vi "Calibrate LCVR.vi"() -> ()   [LabVIEW 2012]
uses:
  <vilib>/DAQmx/write.llb/DAQmx Write (Analog DBL 1Chan 1Samp).vi
  <vilib>/DAQmx/write.llb/DAQmx Write (Digital Bool 1Line 1Point).vi
  <vilib>/DAQmx/write.llb/DAQmx Write (Digital 1D Bool 1Chan 1Samp).vi
  <vilib>/DAQmx/create/channels.llb/DAQmx Create Channel (DO-Digital Output).vi
  <vilib>/DAQmx/create/channels.llb/DAQmx Create Channel (AO-Voltage-Basic).vi
  <vilib>/DAQmx/miscellaneous.llb/DAQmx Fill In Error Info.vi
  <userlib>/metrolib-x86/metrolib-x86.lvlib
panel:
  in  "Ouput Path":path
  in  "Focus":bool
  out "Contrast":cluster{dbl[], dbl[]}(graph)
  out "Image":dbl[][](graph)
  out "Current V":dbl
  out "step":i32
  out "Delta V":dbl
  in  "Steps":i32=40
  in  "Max V":dbl=8.0
  in  "Min V":dbl
  in  "Exposure (ms)":dbl=50.0
  in  "stop":bool
  in  "Sweep":bool
  out "Error Out":errorcluster
  in  "SLM RO":u8 max=38
  # "LCVR Calibration Tool"
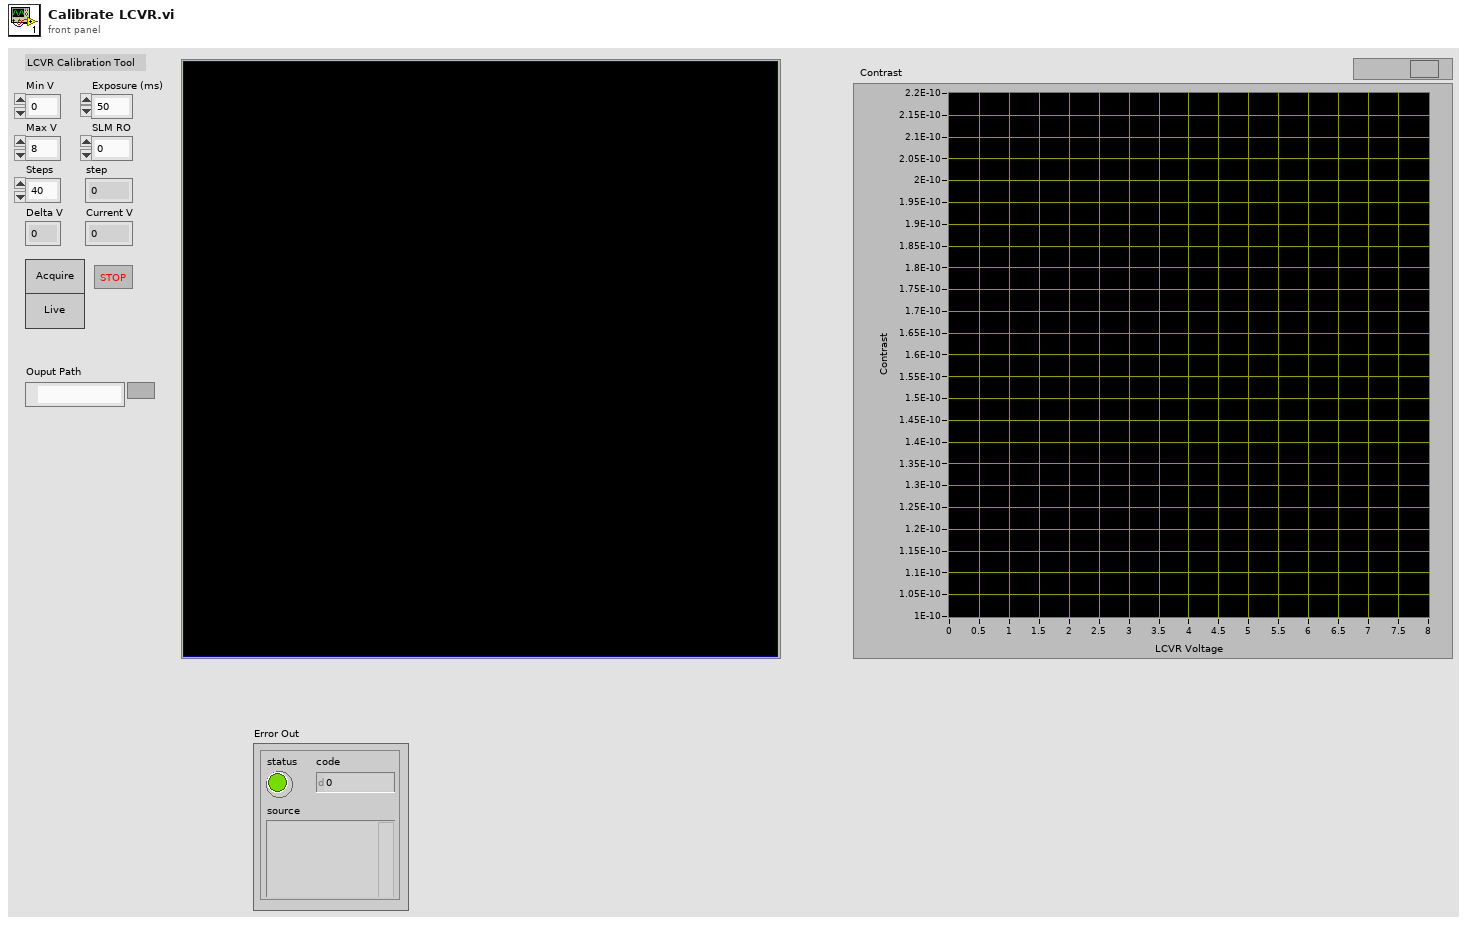
[diagram p1: front panel]
types:
  T1 = cluster{"Mode":u32, "Polarity":u32, "Period":dbl, "Delay":dbl}
  T2 = cluster{"Horizontal Offset":i32, "Vertical Offset":i32, "Horizontal Width":i32, "Vertical Width":i32}
  T3 = cluster{"height":u32, "width":u32, "datatype":u32}
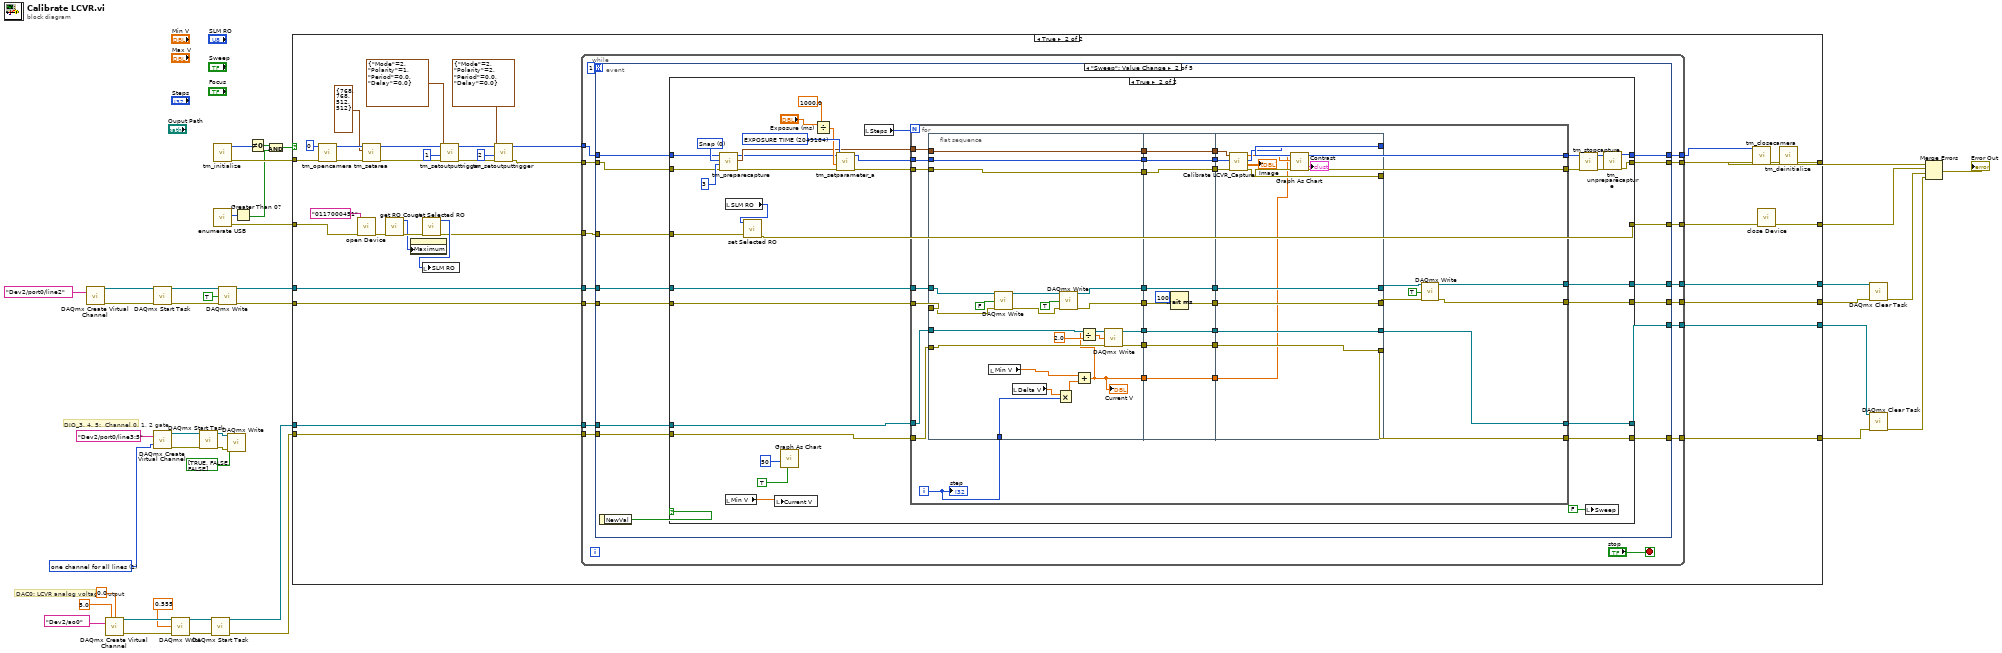
[diagram p0: block diagram]
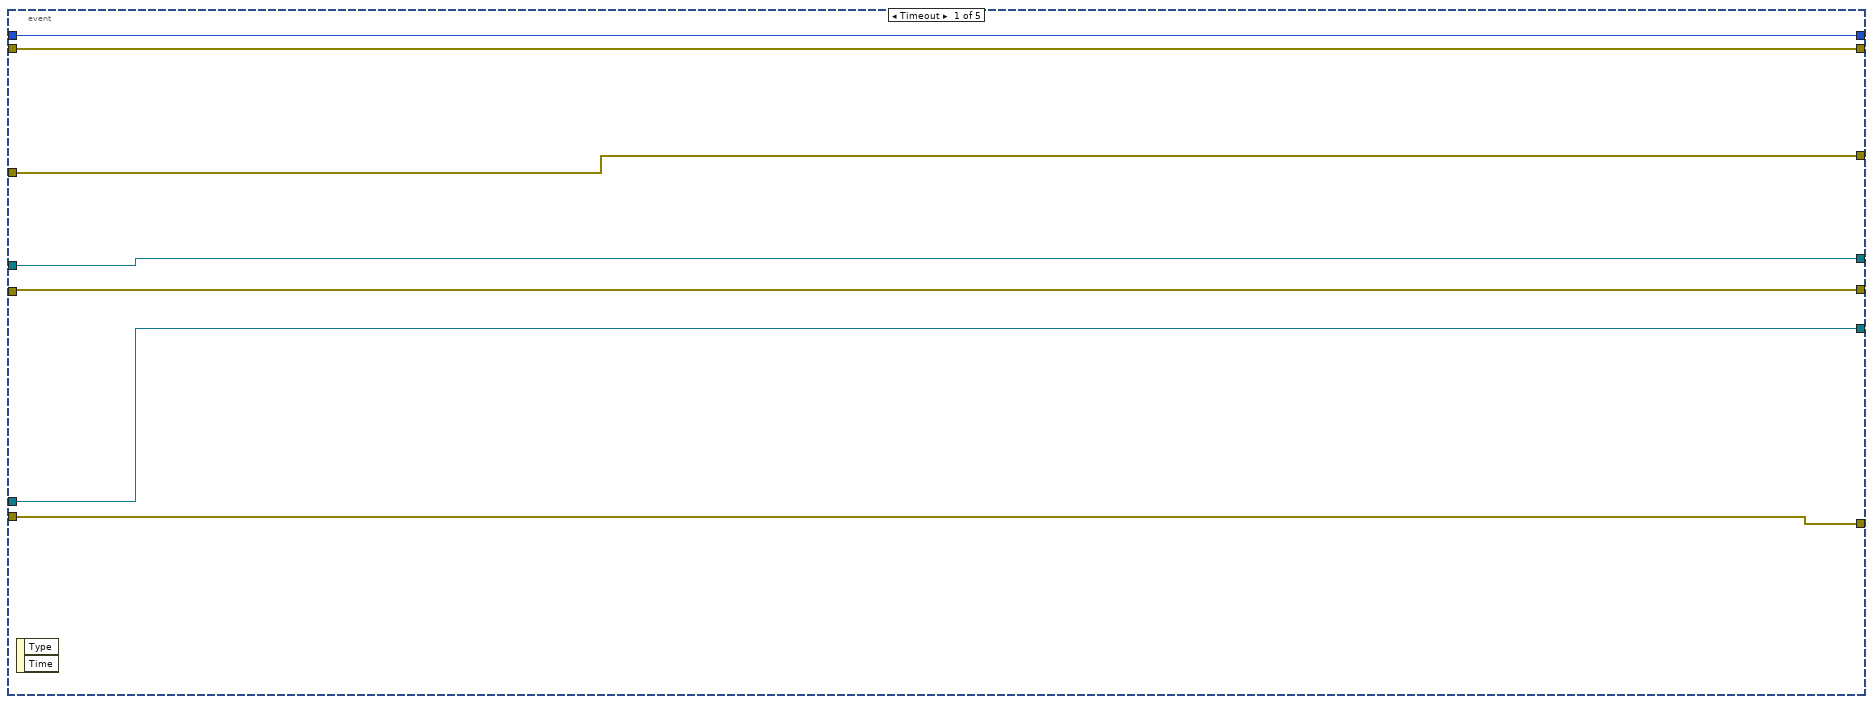
[diagram p3: hidden frame]
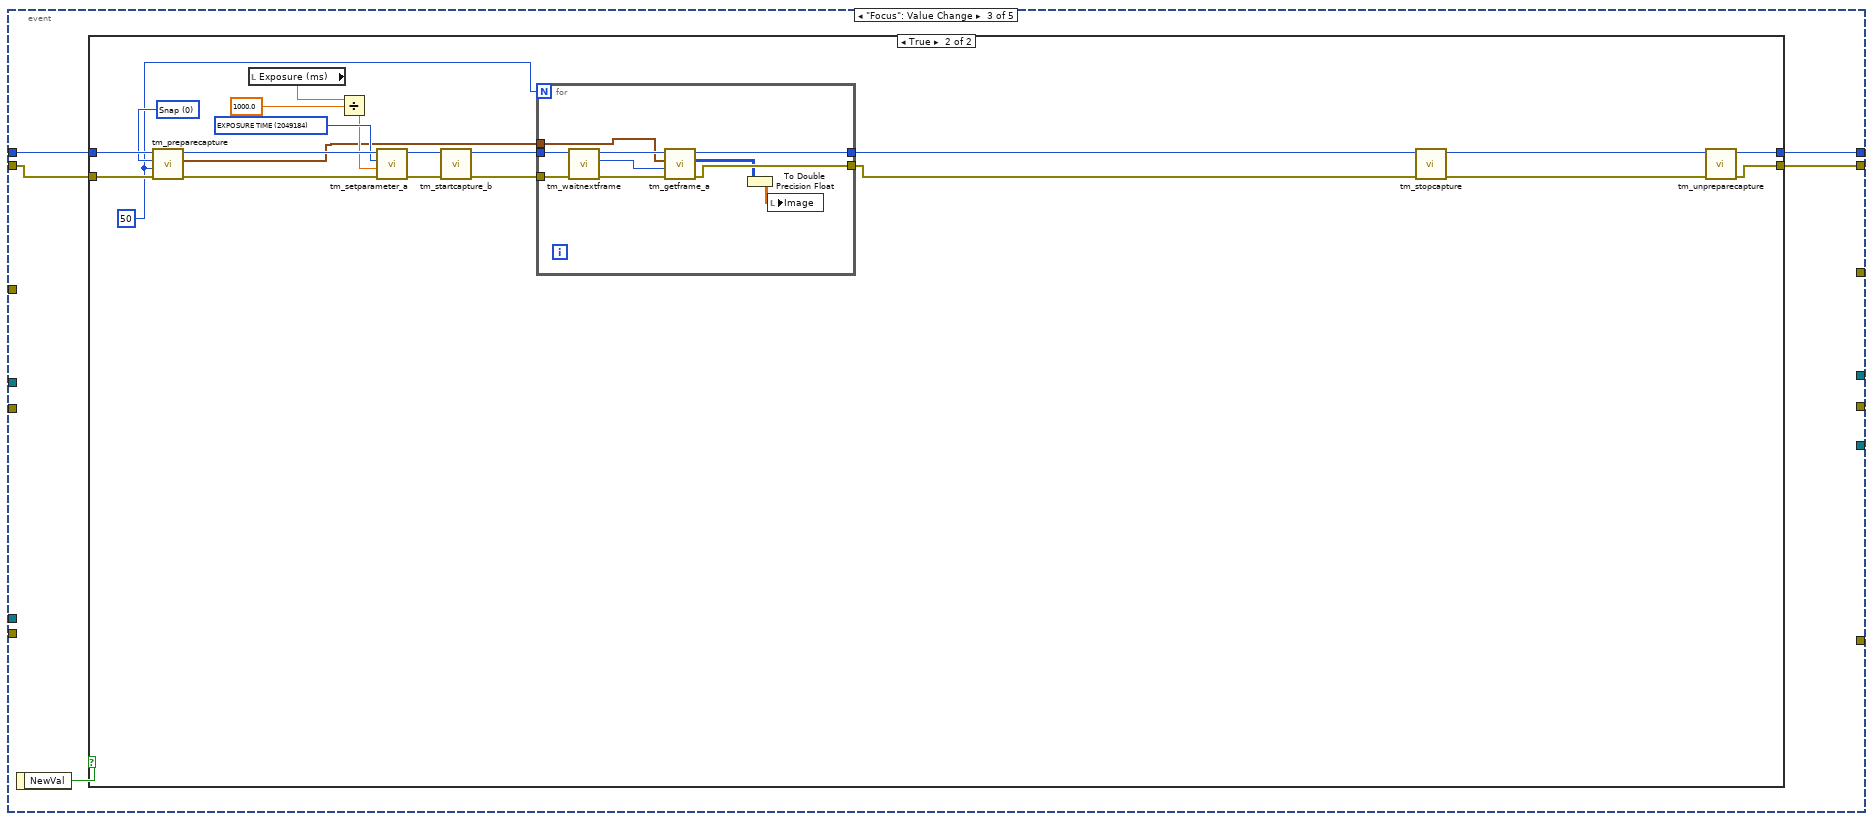
[diagram p5: hidden frame]
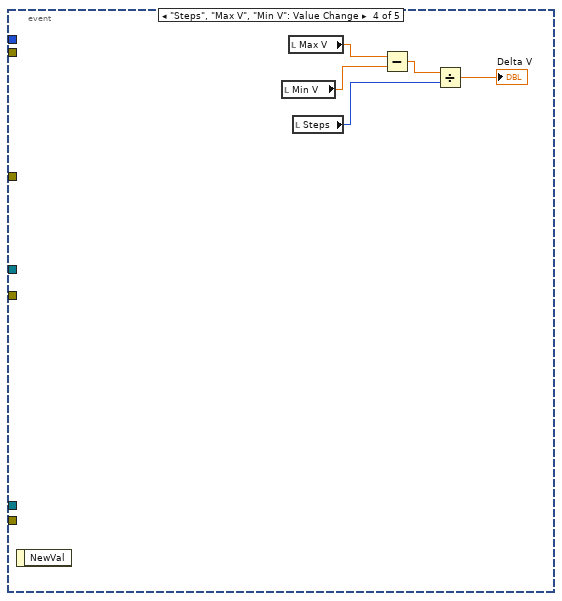
[diagram p7: hidden frame]
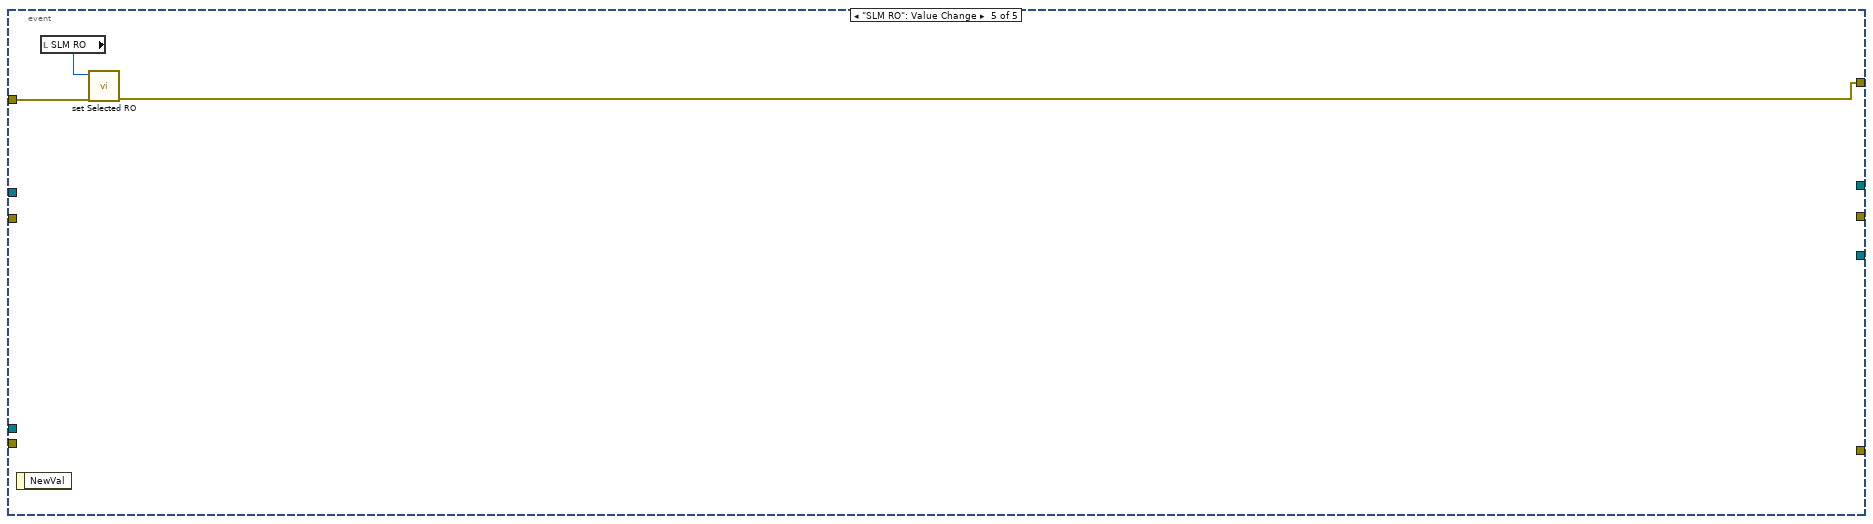
[diagram p8: hidden frame]
diagram:
  w30 = 1 items=["one channel for each line", "one channel for all lines"] ("line grouping")
  # "DAC0: LCVR analog voltage output"
  # "DIO_3, 4, 5:  Channel 0, 1, 2 gate"
  n1 = call-poly <vilib>:"DAQmx Create Virtual Channel.vi"("lines"=tag "Dev2/port0/line2") -> ("task out"=w26:refnum<k21>, "error out"=w25:errorcluster)  [unwired: 13 in]
  n2 = call-poly <vilib>:"DAQmx Create Virtual Channel.vi"("maximum value"=5.0, "minimum value"=0.0, "physical channels"=tag "Dev2/ao0") -> ("task out"=w8:refnum<k21>, "error out"=w7:errorcluster)  [unwired: 11 in]
  n3 = call <vilib>:"DAQmx Start Task.vi"("task/channels in"=w26, "error in"=w25) -> ("task out"=w24:refnum<k21>, "error out"=w23:errorcluster)  [unwired: 12 in]
  n4 = call-poly <vilib>:"DAQmx Create Virtual Channel.vi"("lines"="Dev2/port0/line3:5", "line grouping"=w30) -> ("task out"=w29:refnum<k21>, "error out"=w28:errorcluster)  [unwired: 12 in]
  n5 = call-poly <vilib>:"DAQmx Write.vi"("task/channels in"=w8, "data"=0.555, "error in"=w7) -> ("task out"=w12:refnum<k21>, "error out"=w11:errorcluster)  [unwired: 10 in, 1 out]
  n6 = call <vilib>:"DAQmx Start Task.vi"("task/channels in"=w29, "error in"=w28) -> ("task out"=w21:refnum<k21>, "error out"=w14:errorcluster)  [unwired: 12 in]
  n7 = call <vilib>:"DAQmx Start Task.vi"("task/channels in"=w12, "error in"=w11) -> ("task out"=w4:refnum<k21>, "error out"=w3:errorcluster)  [unwired: 12 in]
  n8 = call <userlib>:"tm_initialize.vi"() -> ("error out"=w39:errorcluster, "Number Of Cameras"=w40:u32)  [unwired: 8 in, 2 out]
  n9 = call <userlib>:"enumerate USB.vi"() -> ("error out"=w38:errorcluster, "function return"=w41:i16)  [unwired: 9 in, 1 out]
  n10 = call-poly <vilib>:"DAQmx Write.vi"("task/channels in"=w24, "data"=TRUE, "error in"=w23) -> ("task out"=w19:refnum<k21>, "error out"=w18:errorcluster)  [unwired: 10 in, 1 out]
  n11 = call-poly <vilib>:"DAQmx Write.vi"("task/channels in"=w21, "data"=bool[] [TRUE, FALSE, FALSE], "error in"=w14) -> ()  [unwired: 10 in, 3 out]
  n12 = Greater Than 0?(x=w41) -> (x > 0?=w35:bool)
  n13 = Not Equal To 0?(x=w40) -> (x != 0?=w37:bool)
  n14 = And(x=w37, y=w35) -> (x .and. y?=w36:bool)
  n15 = case shown="True" w36 {
    tunnel: w39 -> [w47 w82]
    tunnel: w38 -> [w46 w76]
    tunnel: [w47 w73] -> w33
    tunnel: [w46 w71] -> w32
    tunnel: w19 -> [w45 w59]
    tunnel: w18 -> [w44 w58]
    tunnel: [w44 w57] -> w17
    tunnel: [w45 w56] -> w16
    tunnel: w4 -> [w43 w55]
    tunnel: w3 -> [w42 w54]
    tunnel: [w43 w53] -> w2
    tunnel: [w42 w52] -> w1
    frame False {
    }
    frame True {
      n16 = call <userlib>:"tm_opencamera.vi"("error in (no error)"=w82, "Camera Index"=u32 0) -> ("error out"=w70:errorcluster, "Handle out"=w69:u32)  [unwired: 7 in, 1 out]
      n17 = call <userlib>:"open Device.vi"("error in (no error)"=w76, "identifier"="0117000451") -> ("error out"=w77:errorcluster)  [unwired: 8 in, 1 out]
      n18 = call <userlib>:"tm_setarea.vi"("error in (no error)"=w70, "Sub Region"=T2 {"Horizontal Offset"=768, "Vertical Offset"=768, "Horizontal Width"=512, "Vertical Width"=512}, "Handle in"=w69) -> ("error out"=w64:errorcluster, "Handle out"=w67:u32)  [unwired: 7 in]
      n19 = call <userlib>:"get RO Count.vi"("error in (no error)"=w77) -> ("error out"=w79:errorcluster, "count"=w78:u8)  [unwired: 8 in, 1 out]
      n20 = property on="SLM RO" class="DigNum (strict)"("Maximum"=w78) -> ()  [unwired: 2 in, 2 out]
      n21 = call <userlib>:"get Selected RO.vi"("error in (no error)"=w79) -> ("error out"=w75:errorcluster, "selectedRO"=w81:u8)  [unwired: 8 in, 1 out]
      n22 = local write "SLM RO"(w81) -> ()
      n23 = call <userlib>:"tm_setoutputtrigger.vi"("error in (no error)"=w64, "Index"=1, "Parameters"=T1 {"Mode"=2, "Polarity"=1, "Period"=0.0, "Delay"=0.0}, "Handle in"=w67) -> ("error out"=w65:errorcluster, "Handle out"=w66:u32)  [unwired: 6 in]
      n24 = call <userlib>:"tm_setoutputtrigger.vi"("error in (no error)"=w65, "Index"=2, "Parameters"=T1 {"Mode"=2, "Polarity"=2, "Period"=0.0, "Delay"=0.0}, "Handle in"=w66) -> ("error out"=w50:errorcluster, "Handle out"=w51:u32)  [unwired: 6 in]
      n25 = while {
        tunnel: [w99] -> w72
        tunnel: w75 -> [w98]
        tunnel: w50 -> [w97]
        tunnel: [w96] -> w48
        tunnel: [w93] -> w49
        tunnel: w59 -> [w92]
        tunnel: w58 -> [w91]
        tunnel: [w90] -> w57
        tunnel: [w89] -> w56
        tunnel: w55 -> [w88]
        tunnel: w54 -> [w87]
        tunnel: [w86] -> w53
        tunnel: [w85] -> w52
        tunnel: w51 -> [w84]
        stop <- "stop" stop-if-true
        n26 = event shown="[1] \"Sweep\": Value Change" {
          selector: _ -> [_ _ _ _ _]
          dyn-events: _ -> [_ _ _ _ _]
          timeout: 1 -> [_ _ _ _ _]
          tunnel: [w106 w113 _ _ w285] -> w99
          tunnel: w98 -> [w106 w114 _ _ w286]
          tunnel: w97 -> [w105 w107 w243 _ _]
          tunnel: [w105 w119 w242 _ _] -> w96
          tunnel: w84 -> [w104 w108 w244 _ _]
          tunnel: [w104 w120 w241 _ _] -> w93
          tunnel: w92 -> [w103 w118 _ _ _]
          tunnel: w91 -> [w102 w117 _ _ _]
          tunnel: [w102 w116 _ _ _] -> w90
          tunnel: [w103 w115 _ _ _] -> w89
          tunnel: w88 -> [w101 w112 _ _ _]
          tunnel: w87 -> [w100 w111 _ _ _]
          tunnel: [w101 w110 _ _ _] -> w86
          tunnel: [w100 w109 _ _ _] -> w85
          event Timeout {
            n27 = event-data() -> ()  [unwired: 1 in, 2 out]
          }
          event "Sweep": Value Change {
            n28 = event-data() -> ("NewVal"=w121:bool)  [unwired: 1 in]
            n29 = case shown="True" w121 {
              tunnel: w107 -> [w127 w138]
              tunnel: w108 -> [w128 w139]
              tunnel: [w128 w130] -> w120
              tunnel: [w127 w129] -> w119
              tunnel: w118 -> [w126 w148]
              tunnel: w117 -> [w125 w147]
              tunnel: [w125 w145] -> w116
              tunnel: [w126 w146] -> w115
              tunnel: w114 -> [w124 w161]
              tunnel: [w124 w159] -> w113
              tunnel: w112 -> [w123 w152]
              tunnel: w111 -> [w122 w151]
              tunnel: [w123 w150] -> w110
              tunnel: [w122 w149] -> w109
              frame False {
              }
              frame True {
                w140 = 0 items=["Snap", "Sequence"] ("Capture mode")
                w162 = u32 2049184 items=["SENSOR MODE"=4212128, "CCD MODE"=4212384, "READOUT MODE"=4211872, "ACTIVE VIEW INDEX"=4343136, "BITS PER CHANNEL"=4342976, "IMAGE PIXEL TYPE"=4343296, "BINNING"=4215968, "EXPOSURE TIME"=2049184, "CONTRAST GAIN"=3163312, "CONTRAST OFFSET"=3163328, "LIGHT MODE"=2114720, "SENSITIVITY"=2114992, "PHOTON IMAGING MODE"=2115200, "HIGH DYNAMIC RANGE MODE"=3163360, "WHITE BALANCE"=3163568, "TEMPERATURE"=2115232, "TEMPERATURE TARGET"=2115264, "SENSOR COOLER FAN"=2115296, "LINEBUNDLE HEIGHT"=4212192, "MECHANICAL SHUTTER"=2115488, "BACK FOCUS POSITION"=8422304, "TRIGGER CONNECTOR"=1066432, "TRIGGER SOURCE"=1066144, "OUTPUT TRIGGER SOURCE"=1852576, "TRIGGER GLOBAL EXPOSURE"=2049680, "FIRST TRIGGER BEHAVIOR"=2049696, "CHANNEL SYNC"=1852352, "READOUT DIRECTION"=4211904, "PRE HSYNC COUNT"=1852704, "INTERNAL LINE SPEED"=4226000, "INTERNAL LINE INTERVAL"=4226016] ("Parameter")
                n30 = call <userlib>:"tm_preparecapture.vi"("error in (no error)"=w138, "Frames"=3, "Capture mode"=w140, "Handle in"=w139) -> ("error out"=w137:errorcluster, "Buffer Info"=w136:T3, "Handle out"=w135:u32)  [unwired: 4 in, 1 out]
                n31 = local read "SLM RO"() -> (w160:u8)
                n32 = local read "Min V"() -> (w144:dbl)
                n33 = call <userlib>:"set Selected RO.vi"("error in (no error)"=w161, "runningOrder"=w160) -> ("error out"=w159:errorcluster)  [unwired: 8 in, 1 out]
                n34 = local write "Current V"(w144) -> ()
                n35 = call "Graph As Chart.vi"("Clear Graph?"=TRUE, "Chart History (10,000)"=50) -> ()  [unwired: 9 in, 1 out]
                n36 = Divide(x="Exposure (ms)", y=1000.0) -> (x/y=w157:dbl)
                n37 = call <userlib>:"tm_setparameter_a.vi"("error in (no error)"=w137, "Value in"=w157, "Parameter"=w162, "Handle in"=w135) -> ("error out"=w154:errorcluster, "Handle out"=w155:u32)  [unwired: 6 in]
                n38 = local read "Steps"() -> (w153:i32)
                n39 = for {
                  N: w153 -> [_]
                  tunnel: w136 -> [w183]
                  tunnel: w155 -> [w182]
                  tunnel: w154 -> [w179]
                  tunnel: [w176] -> w134
                  tunnel: [w175] -> w133
                  tunnel: w152 -> [w174]
                  tunnel: w151 -> [w173]
                  tunnel: [w172] -> w150
                  tunnel: [w169] -> w149
                  tunnel: w148 -> [w187]
                  tunnel: w147 -> [w186]
                  tunnel: [w193] -> w146
                  tunnel: [w192] -> w145
                  i -> [w164]
                  n40 = flat-sequence {
                    tunnel: [w218] -> w189
                    tunnel: [w217] -> w188
                    tunnel: w187 -> [w200]
                    tunnel: w186 -> [w199]
                    tunnel: [w215] -> w184
                    tunnel: w183 -> [w215]
                    tunnel: w182 -> [w214]
                    tunnel: [w214] -> w181
                    tunnel: w179 -> [w213]
                    tunnel: [w213] -> w178
                    tunnel: w174 -> [w207]
                    tunnel: w173 -> [w206]
                    tunnel: [w205] -> w170
                    tunnel: [w204] -> w167
                    tunnel: [w203] -> w165
                    tunnel: w164 -> [w202]
                    tunnel: [w227] -> w191
                    tunnel: [w226] -> w190
                    tunnel: w189 -> [w226]
                    tunnel: w188 -> [w227]
                    tunnel: [w224] -> w185
                    tunnel: w184 -> [w224]
                    tunnel: w181 -> [w223]
                    tunnel: [w223] -> w180
                    tunnel: w178 -> [w222]
                    tunnel: [w222] -> w177
                    tunnel: [w221] -> w171
                    tunnel: w170 -> [w221]
                    tunnel: [w220] -> w168
                    tunnel: w167 -> [w220]
                    tunnel: [w219] -> w166
                    tunnel: w165 -> [w219]
                    tunnel: [w239] -> w196
                    tunnel: [w240] -> w195
                    tunnel: w191 -> [w240]
                    tunnel: w190 -> [w239]
                    tunnel: w185 -> [w236]
                    tunnel: w180 -> [w235]
                    tunnel: w177 -> [w234]
                    tunnel: [w233] -> w176
                    tunnel: [w232] -> w175
                    tunnel: [w231] -> w172
                    tunnel: w171 -> [w231]
                    tunnel: [w230] -> w169
                    tunnel: w168 -> [w230]
                    tunnel: w166 -> [w228]
                    frame #0 {
                      n41 = local read "Min V"() -> (w209:dbl)
                      n42 = call-poly <vilib>:"DAQmx Write.vi"("task/channels in"=w200, "data"=FALSE, "error in"=w199) -> ("task out"=w198:refnum<k21>, "error out"=w197:errorcluster)  [unwired: 10 in, 1 out]
                      n43 = local read "Delta V"() -> (w208:dbl)
                      n44 = Multiply(x=w208, y=w202) -> (x*y=w212:dbl)
                      n45 = call-poly <vilib>:"DAQmx Write.vi"("task/channels in"=w198, "data"=TRUE, "error in"=w197) -> ("task out"=w218:refnum<k21>, "error out"=w217:errorcluster)  [unwired: 10 in, 1 out]
                      n46 = Add(x=w209, y=w212) -> (x+y=w203:dbl)
                      "Current V" <- w203
                      n47 = Divide(x=w203, y=2.0) -> (x/y=w210:dbl)
                      n48 = call-poly <vilib>:"DAQmx Write.vi"("task/channels in"=w207, "data"=w210, "error in"=w206) -> ("task out"=w205:refnum<k21>, "error out"=w204:errorcluster)  [unwired: 10 in, 1 out]
                    }
                    frame #1 {
                      n49 = Wait (ms)(milliseconds to wait=u32 100) -> ()  [unwired: 1 out]
                    }
                    frame #2 {
                      n50 = call "Calibrate LCVR_Capture.vi"("error in (no error)"=w234, "Handle in"=w235, "Buffer Info"=w236) -> ("error out"=w232:errorcluster, "Image"=→"Image":dbl[][], "Handle out"=w233:u32, "contrast"=w229:dbl)  [unwired: 5 in]
                      n51 = call "Graph As Chart.vi"("Y Value"=w229, "X Value"=w228) -> ("XY Graph"=→"Contrast":cluster{dbl[], dbl[]})  [unwired: 9 in]
                    }
                  }
                  n52 = call-poly <vilib>:"DAQmx Write.vi"("task/channels in"=w196, "data"=TRUE, "error in"=w195) -> ("task out"=w193:refnum<k21>, "error out"=w192:errorcluster)  [unwired: 10 in, 1 out]
                  "step" <- w164
                }
                n53 = call <userlib>:"tm_stopcapture.vi"("error in (no error)"=w133, "Handle in"=w134) -> ("error out"=w131:errorcluster, "Handle out"=w132:u32)  [unwired: 8 in]
                n54 = local write "Sweep"(FALSE ("Snap")) -> ()
                n55 = call <userlib>:"tm_unpreparecapture.vi"("error in (no error)"=w131, "Handle in"=w132) -> ("error out"=w129:errorcluster, "Handle out"=w130:u32)  [unwired: 8 in]
              }
            }
          }
          event "Focus": Value Change {
            n56 = event-data() -> ("NewVal"=w245:bool)  [unwired: 1 in]
            n57 = case shown="True" w245 {
              tunnel: w244 -> [w247 w268]
              tunnel: w243 -> [w246 w267]
              tunnel: [w246 w248] -> w242
              tunnel: [w247 w249] -> w241
              frame False {
              }
              frame True {
                w254 = 50 ("Frames")
                w263 = u32 2049184 items=["SENSOR MODE"=4212128, "CCD MODE"=4212384, "READOUT MODE"=4211872, "ACTIVE VIEW INDEX"=4343136, "BITS PER CHANNEL"=4342976, "IMAGE PIXEL TYPE"=4343296, "BINNING"=4215968, "EXPOSURE TIME"=2049184, "CONTRAST GAIN"=3163312, "CONTRAST OFFSET"=3163328, "LIGHT MODE"=2114720, "SENSITIVITY"=2114992, "PHOTON IMAGING MODE"=2115200, "HIGH DYNAMIC RANGE MODE"=3163360, "WHITE BALANCE"=3163568, "TEMPERATURE"=2115232, "TEMPERATURE TARGET"=2115264, "SENSOR COOLER FAN"=2115296, "LINEBUNDLE HEIGHT"=4212192, "MECHANICAL SHUTTER"=2115488, "BACK FOCUS POSITION"=8422304, "TRIGGER CONNECTOR"=1066432, "TRIGGER SOURCE"=1066144, "OUTPUT TRIGGER SOURCE"=1852576, "TRIGGER GLOBAL EXPOSURE"=2049680, "FIRST TRIGGER BEHAVIOR"=2049696, "CHANNEL SYNC"=1852352, "READOUT DIRECTION"=4211904, "PRE HSYNC COUNT"=1852704, "INTERNAL LINE SPEED"=4226000, "INTERNAL LINE INTERVAL"=4226016] ("Parameter")
                w266 = 0 items=["Snap", "Sequence"] ("Capture mode")
                n58 = call <userlib>:"tm_preparecapture.vi"("error in (no error)"=w267, "Frames"=w254, "Capture mode"=w266, "Handle in"=w268) -> ("error out"=w264:errorcluster, "Buffer Info"=w255:T3, "Handle out"=w265:u32)  [unwired: 4 in, 1 out]
                n59 = local read "Exposure (ms)"() -> (w261:dbl)
                n60 = Divide(x=w261, y=1000.0) -> (x/y=w262:dbl)
                n61 = call <userlib>:"tm_setparameter_a.vi"("error in (no error)"=w264, "Value in"=w262, "Parameter"=w263, "Handle in"=w265) -> ("error out"=w258:errorcluster, "Handle out"=w259:u32)  [unwired: 6 in]
                n62 = call <userlib>:"tm_startcapture_b.vi"("error in (no error)"=w258, "Handle in"=w259) -> ("error out"=w256:errorcluster, "Handle out"=w257:u32)  [unwired: 8 in]
                n63 = for {
                  N: w254 -> [_]
                  tunnel: w257 -> [w278]
                  tunnel: w256 -> [w277]
                  tunnel: w255 -> [w275]
                  tunnel: [w273] -> w253
                  tunnel: [w272] -> w252
                  n64 = call <userlib>:"tm_waitnextframe.vi"("error in (no error)"=w277, "Handle in"=w278) -> ("error out"=w274:errorcluster, "Frame Index"=w269:i32, "Handle out"=w276:u32)  [unwired: 6 in, 1 out]
                  n65 = call <userlib>:"tm_getframe_a.vi"("error in (no error)"=w274, "Frame Index"=w269, "Buffer Info"=w275, "Handle in"=w276) -> ("error out"=w272:errorcluster, "Data 16"=w271:u16[][], "Handle out"=w273:u32)  [unwired: 3 in, 2 out]
                  n66 = To Double Precision Float(number=w271) -> (double precision float=w270:dbl[][])
                  n67 = local write "Image"(w270) -> ()
                }
                n68 = call <userlib>:"tm_stopcapture.vi"("error in (no error)"=w252, "Handle in"=w253) -> ("error out"=w250:errorcluster, "Handle out"=w251:u32)  [unwired: 8 in]
                n69 = call <userlib>:"tm_unpreparecapture.vi"("error in (no error)"=w250, "Handle in"=w251) -> ("error out"=w248:errorcluster, "Handle out"=w249:u32)  [unwired: 8 in]
              }
            }
          }
          event "Steps", "Max V", "Min V": Value Change {
            n70 = event-data() -> ()  [unwired: 1 in, 1 out]
            n71 = local read "Min V"() -> (w282:dbl)
            n72 = local read "Max V"() -> (w283:dbl)
            n73 = local read "Steps"() -> (w280:i32)
            n74 = Subtract(x=w283, y=w282) -> (x-y=w281:dbl)
            n75 = Divide(x=w281, y=w280) -> (x/y=→"Delta V":dbl)
          }
          event "SLM RO": Value Change {
            n76 = event-data() -> ()  [unwired: 1 in, 1 out]
            n77 = local read "SLM RO"() -> (w284:u8)
            n78 = call <userlib>:"set Selected RO.vi"("error in (no error)"=w286, "runningOrder"=w284) -> ("error out"=w285:errorcluster)  [unwired: 8 in, 1 out]
          }
        }
      }
      n79 = call <userlib>:"tm_closecamera.vi"("error in (no error)"=w48, "Handle in"=w49) -> ("error out"=w74:errorcluster)  [unwired: 9 in]
      n80 = call <userlib>:"close Device.vi"("error in (no error)"=w72) -> ("error out"=w71:errorcluster)  [unwired: 9 in, 1 out]
      n81 = call <userlib>:"tm_deinitialize.vi"("error in (no error)"=w74) -> ("error out"=w73:errorcluster)  [unwired: 10 in]
    }
  }
  n82 = call <vilib>:"DAQmx Clear Task.vi"("task in"=w16, "error in"=w17) -> ("error out"=w15:errorcluster)  [unwired: 13 in]
  n83 = call <vilib>:"DAQmx Clear Task.vi"("task in"=w2, "error in"=w1) -> ("error out"=w5:errorcluster)  [unwired: 13 in]
  n84 = Merge Errors(w33, w32, w15, w5) -> (→"Error Out":errorcluster)
